vi "ICRA2024没有ratio控制只有轨迹跟踪.vi"() -> ()   [LabVIEW 2018]
doc: "Demonstrates the use of the Network Streams functions to send LED status to the myRIO target."
uses:
  <vilib>/Utility/file.llb/Read Delimited Spreadsheet (string).vi
  <vilib>/ErrorRing/Error Ring.xnode
  <vilib>/vision/NI_Vision_Development_Module.lvlib
panel:
  out "轨迹跟踪点数":i32[](array[numeric])
  out "数据总":dbl[][](array[numeric])
  out "时间T":i32[](array[numeric])
  out "运动方向":sgl[](array[numeric])
  out "aspectratio":dbl[](array[numeric])
  in  "轨迹打开":bool
  out "实际纵坐标":sgl
  out "实际横坐标":sgl
  out "方向d1":sgl
  out "轨迹跟踪点数":i32
  out "目标点y":dbl
  out "目标点x":dbl
  out "b":dbl[](array[numeric])
  in  "pp":dbl
  out "与目标点的距离":sgl
  in  "guiji":path=path "D:/lyz/ICRA2024-YuezhenLiu/small_myRIO_Helmholtz - 1111ke777/zgj轨迹跟踪只有20个点.txt" caption="call7-8"
  out "裁剪后的二值图":T1(plugin-control)
  in  "布尔":bool
  in  "ribbon磁场开关":bool=TRUE
  out "面积":sgl
  out "field ratio":sgl=4.0
  out "时间":i32
  out "aspect ratio":dbl
  out "D2":i32
  out "D1":i32
  out "二值图":T1(plugin-control)
  in  "Search Rect (entire image)":T2={"Left"=200, "Top"=120, "Right"=2000, "Bottom"=1920, "Rotation"=0.0} {"Rotation" format="%.2f"; "Left" scale=0.0..1024.0; "Right" scale=0.0..1024.0}
  out "备用的椭圆角度":sgl
  in  "Number of Erosion":i32=10
  out "Image 7":T1(plugin-control)
  in  "Acquisition Control::Acquisition Frame Rate":dbl=19.50304412841797 min=1.4211589097976685 max=44.94382095336914
  out "Stopped":bool
  in  "Stop (F) 2":bool caption="Stop (F)"
  out "Objects 2":T3(array[cluster]) {"Aspect Ratio" format="%.2f"; "Orientation" format="%.2f"; "Area" format="%.2f"; "Object Center"."Y" format="%.2f"; "Object Center"."X" format="%.2f"}
  in  "Settings 2":T4={"Objects"=0, "Threshold"=128, "Reject Border"=FALSE, "Fill Holes"=FALSE, "Min Object Size"=FALSE, "Min Size"=20000, "Max Object Size"=FALSE, "Max Size"=100, "Show Search Area"=FALSE, "Show Center"=TRUE, "Show Bounding Box"=TRUE} {"Objects" items=["Bright Objects", "Dark Objects"]; "Threshold" min=1 max=999999999 step=1; "Max Size" min=1 max=999999999 step=1; "Min Size" min=1 max=999999999 step=1}
  in  "Range 2":cluster{"Lower value":sgl, "Upper value":sgl}={"Lower value"=0.0, "Upper value"=230.0} {"Upper value" format="%.2f"; "Lower value" format="%.2f"}
  in  "Pause":bool
  out "Array":dbl[](array[numeric])
  in  "Parameter Settings":T5(tab)=enum."Ribbon Oscillating Field" caption="Field Types"
  in  "fg":dbl
  in  "pg":dbl
  in  "dg":dbl
  in  "Ag":dbl
  in  "AoOF":dbl
  in  "fo":sgl
  in  "do":sgl
  in  "oo":sgl
  in  "po":sgl
  in  "cc":sgl
  in  "pc":sgl
  in  "wc":sgl
  in  "dc":sgl
  in  "Ac":dbl
  in  "pr":sgl
  in  "Ar":dbl=8.0
  in  "wr":sgl=18.0
  in  "dr":sgl
  in  "Dis phase step":dbl
  in  "Dis phase frequency (Hz)":dbl
  in  "Dis tumbling frequency (Hz)":dbl
  in  "Dis strength(mT)":dbl
  in  "Swa strength (mT)":dbl
  in  "Swa frequency (Hz)":dbl
  in  "Swa pitch angle (deg)":dbl
  in  "Swa direction angle (deg)":dbl
  in  "Swa ratio":dbl=1.0
  in  "Pitch Angle (rotating around Constant, deg)":dbl
  in  "Ratio (A/C)":sgl=4.0
  in  "Direction Angle (deg)":sgl
  in  "Pitch Angle (rotating around Origin, deg)":sgl
  in  "Frequency (Hz)":sgl=10.0
  in  "Strength (mT)":dbl=10.0
  in  "Ar 2":dbl=5.0 caption="Ar"
  in  "ratio":sgl=1.0
  in  "运动方向":sgl
  in  "长轴方向":sgl
  in  "wr  2":sgl=8.0
  in  "速度大小":sgl
  out "Numeric 5":i32
  in  "Stop":bool
  out "error out":errorcluster
  in  "Target IP Address":string="172.22.11.2"
  # "Overview: Magnetic field calculation, and send parameters to myRIO\nInstructions:\n1. Verify the value of Target IP Address. Set Visa resource name.\n2. Ensure RT Main.vi is already running. \n3. Run this VI. Set parameters of magnetic field."
  # "Strength (mT)"
  # "Pitch Angle (deg)"
  # "Direction Angle (deg)"
  # "Frequency (Hz)"
  # "Strength (mT)"
  # "Oscilation Frequency (Hz)"
  # "Oscilation Angle (deg)"
  # "Pitch Angle (deg)"
  # "Direction Angle (deg)"
  # "Strength (mT)"
  # "Frequency (Hz)"
  # "Pitch Angle (deg)"
  # "Direction Angle (deg)"
  # "Conical Angle (deg)"
  # "Strength (mT)"
  # "Frequency (Hz)"
  # "Pitch Angle (deg)"
  # "Direction Angle (deg)"
  # "Strength (mT)"
  # "Tumbling Frequency (Hz)"
  # "Phase Frequency (Hz)"
  # "Phase Step"
  # "Strength (mT)"
  # "Frequency (Hz)"
  # "Pitch Angle (deg)"
  # "Direction Angle (deg)"
  # "Ratio"
  # "Strength (mT)"
  # "Frequency (Hz)"
  # "Ratio (A/C)"
  # "Direction Angle (deg)"
  # "Pitch Angle (rotating around Origin, deg)"
  # "Pitch Angle (rotating around Constant, deg)"
  # "Strength (mT)"
  # "Frequency (Hz)"
  # "Pitch Angle  (deg)"
  # "longaxis"
  # "Direction Angle (deg)"
  # "ratio (l/s)"
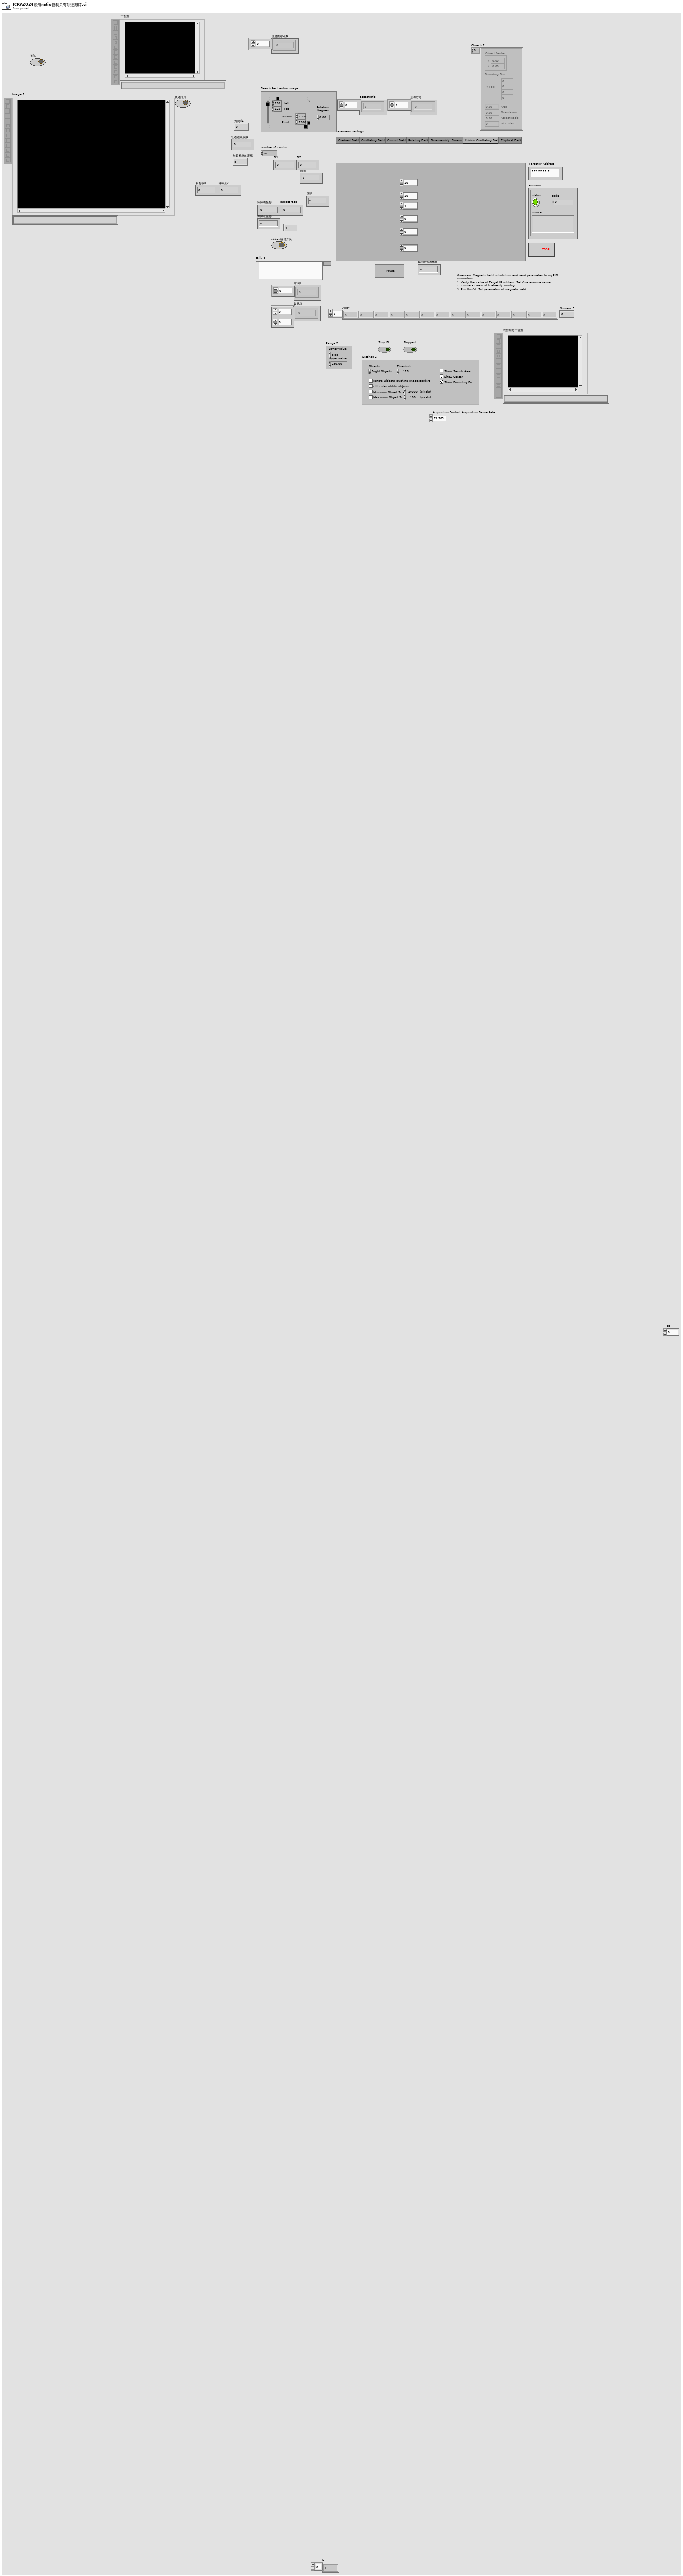
[diagram p1: front panel]
types:
  T1 = typedef "IMAQ Image.ctl" = refnum<image>
  T2 = typedef "IMAQ Rectangle" = cluster{"Left":i32, "Top":i32, "Right":i32, "Bottom":i32, "Rotation":dbl}
  T3 = cluster{"Object Center":cluster{"X":sgl, "Y":sgl}, "Bounding Box":cluster{"X Left":i32, "Y Top":i32, "X Right":i32, "Y Bottom":i32}, "Area":sgl, "Orientation":sgl, "Aspect Ratio":sgl, "Nb Holes":i32}[]
  T4 = cluster{"Objects":u16, "Threshold":i32, "Reject Border":bool, "Fill Holes":bool, "Min Object Size":bool, "Min Size":i32, "Max Object Size":bool, "Max Size":i32, "Show Search Area":bool, "Show Center":bool, "Show Bounding Box":bool}
  T5 = enum32{"Gradient Field ", "Oscillating Field", "Conical Field", "Rotating Field", "Disassembly", "Swarm", "Ribbon Oscillating Field", "Elliptical Field"}
  T6 = typedef "Image Type" = u32
  T7 = cluster{"Objects[0]":cluster{"Object Center":cluster{"X":sgl, "Y":sgl}, "Bounding Box":cluster{"X Left":i32, "Y Top":i32, "X Right":i32, "Y Bottom":i32}, "Area":sgl, "Orientation":sgl, "Aspect Ratio":sgl, "Nb Holes":i32}, "Objects[1]":cluster{"Object Center":cluster{"X":sgl, "Y":sgl}, "Bounding Box":cluster{"X Left":i32, "Y Top":i32, "X Right":i32, "Y Bottom":i32}, "Area":sgl, "Orientation":sgl, "Aspect Ratio":sgl, "Nb Holes":i32}, "Objects[2]":cluster{"Object Center":cluster{"X":sgl, "Y":sgl}, "Bounding Box":cluster{"X Left":i32, "Y Top":i32, "X Right":i32, "Y Bottom":i32}, "Area":sgl, "Orientation":sgl, "Aspect Ratio":sgl, "Nb Holes":i32}, "Objects[3]":cluster{"Object Center":cluster{"X":sgl, "Y":sgl}, "Bounding Box":cluster{"X Left":i32, "Y Top":i32, "X Right":i32, "Y Bottom":i32}, "Area":sgl, "Orientation":sgl, "Aspect Ratio":sgl, "Nb Holes":i32}, "Objects[4]":cluster{"Object Center":cluster{"X":sgl, "Y":sgl}, "Bounding Box":cluster{"X Left":i32, "Y Top":i32, "X Right":i32, "Y Bottom":i32}, "Area":sgl, "Orientation":sgl, "Aspect Ratio":sgl, "Nb Holes":i32}, "Objects[5]":cluster{"Object Center":cluster{"X":sgl, "Y":sgl}, "Bounding Box":cluster{"X Left":i32, "Y Top":i32, "X Right":i32, "Y Bottom":i32}, "Area":sgl, "Orientation":sgl, "Aspect Ratio":sgl, "Nb Holes":i32}, "Objects[6]":cluster{"Object Center":cluster{"X":sgl, "Y":sgl}, "Bounding Box":cluster{"X Left":i32, "Y Top":i32, "X Right":i32, "Y Bottom":i32}, "Area":sgl, "Orientation":sgl, "Aspect Ratio":sgl, "Nb Holes":i32}, "Objects[7]":cluster{"Object Center":cluster{"X":sgl, "Y":sgl}, "Bounding Box":cluster{"X Left":i32, "Y Top":i32, "X Right":i32, "Y Bottom":i32}, "Area":sgl, "Orientation":sgl, "Aspect Ratio":sgl, "Nb Holes":i32}, "Objects[8]":cluster{"Object Center":cluster{"X":sgl, "Y":sgl}, "Bounding Box":cluster{"X Left":i32, "Y Top":i32, "X Right":i32, "Y Bottom":i32}, "Area":sgl, "Orientation":sgl, "Aspect Ratio":sgl, "Nb Holes":i32}}
  T8 = cluster{"Object Center":cluster{"X":sgl, "Y":sgl}, "Bounding Box":cluster{"X Left":i32, "Y Top":i32, "X Right":i32, "Y Bottom":i32}, "Area":sgl, "Orientation":sgl, "Aspect Ratio":sgl, "Nb Holes":i32}
  T9 = cluster{"X Left":i32, "Y Top":i32, "X Right":i32, "Y Bottom":i32}
  T10 = typedef "ROI Descriptor" = cluster{"Global Rectangle":i32[], "Contours":cluster{"ID":enum32{"External", "Internal"}, "Type":u32, "Coordinates":i32[]}[]}
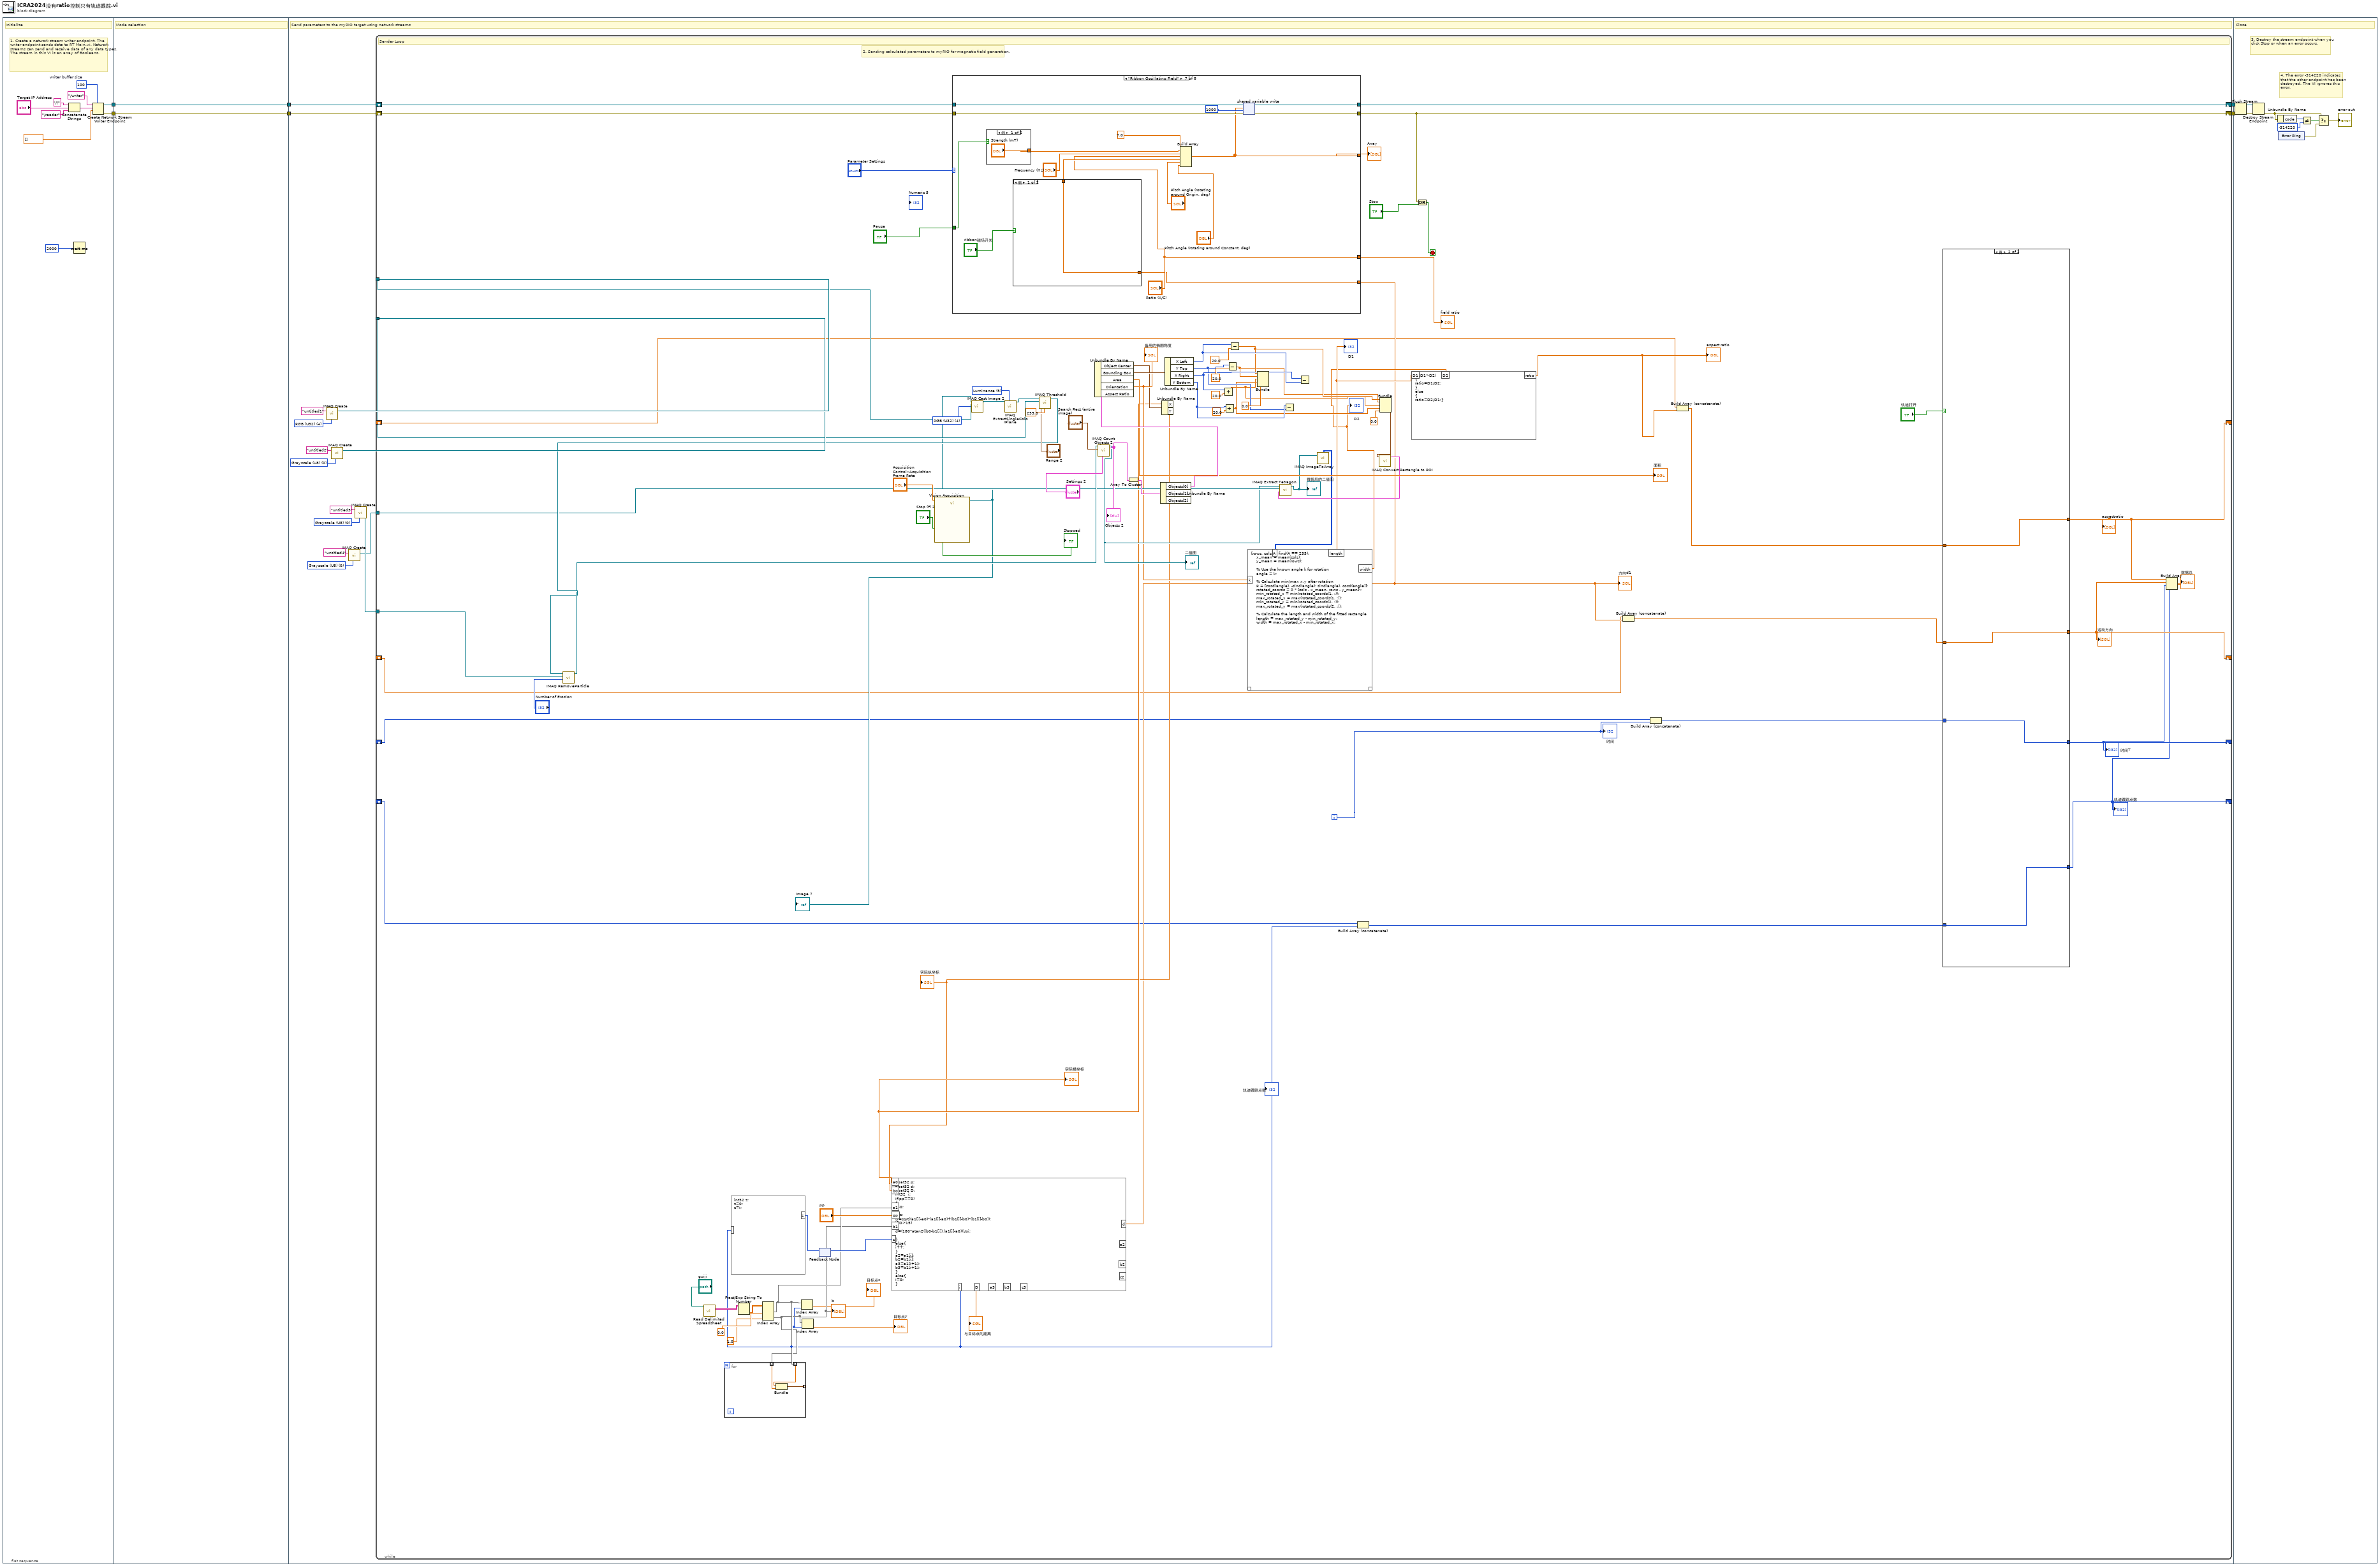
[diagram p0: block diagram]
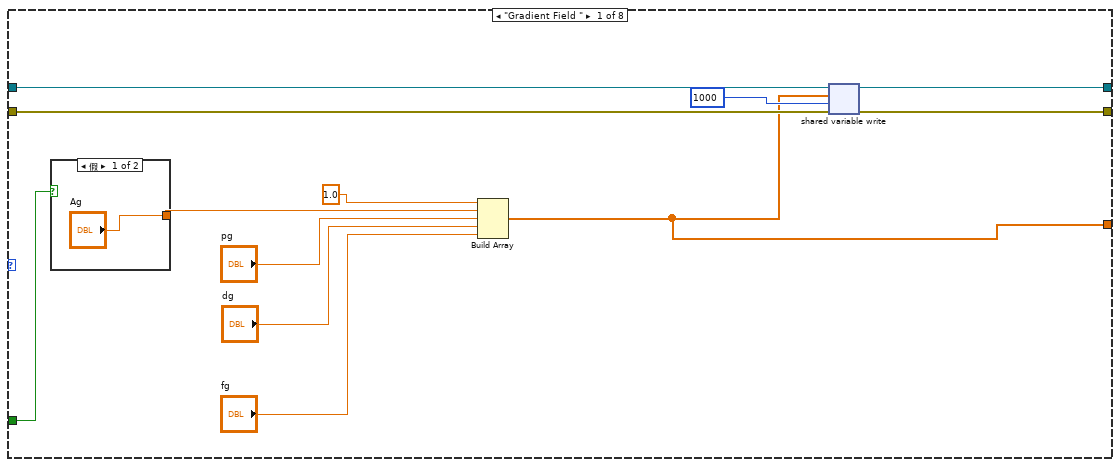
[diagram p3: hidden frame]
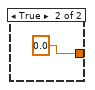
[diagram p4: hidden frame]
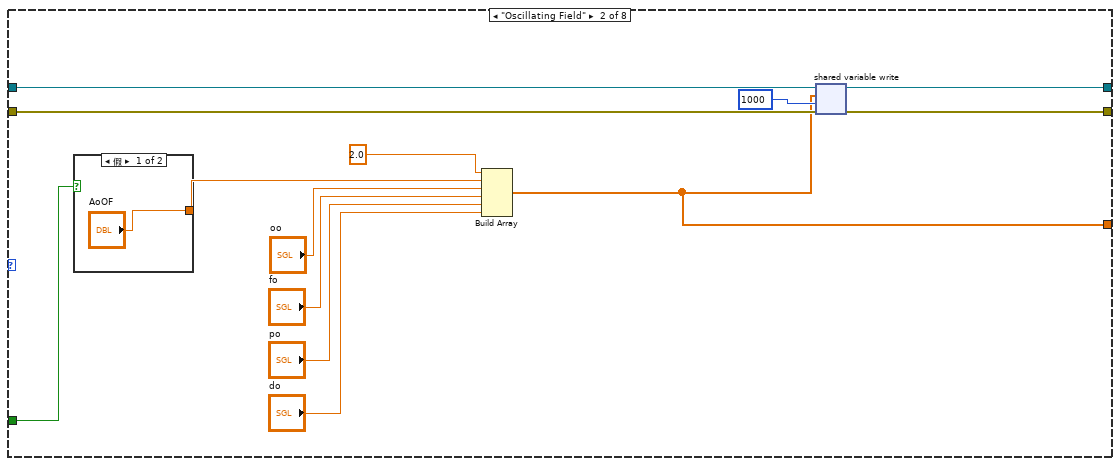
[diagram p5: hidden frame]
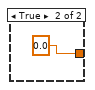
[diagram p6: hidden frame]
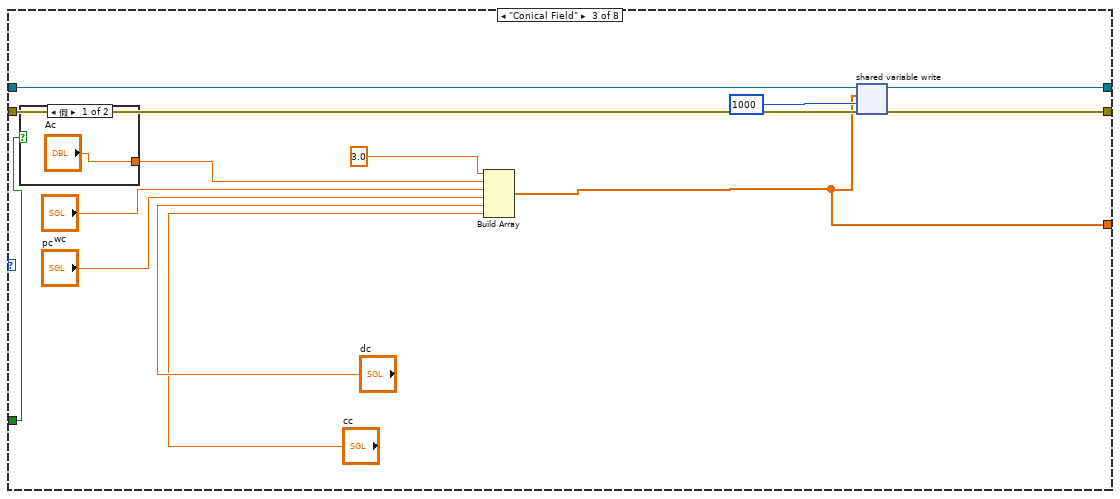
[diagram p7: hidden frame]
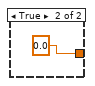
[diagram p8: hidden frame]
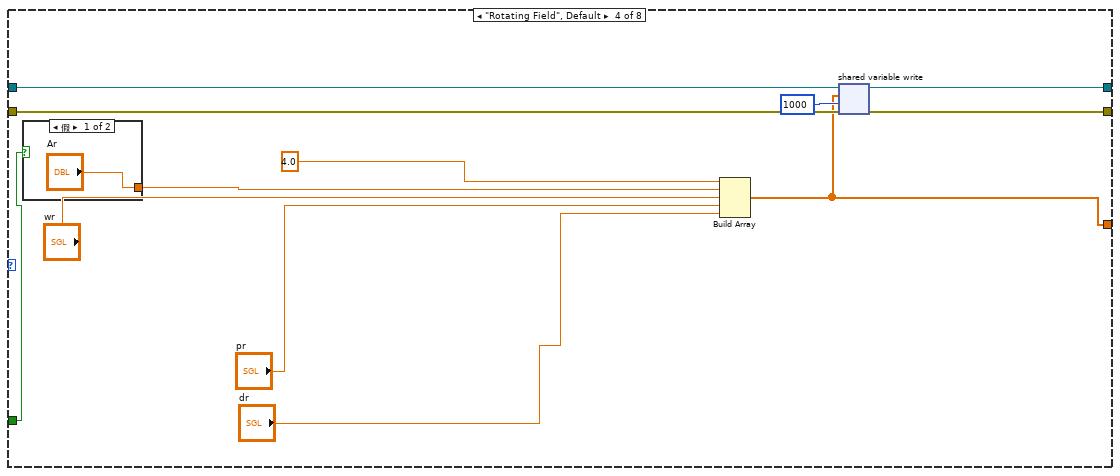
[diagram p9: hidden frame]
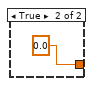
[diagram p10: hidden frame]
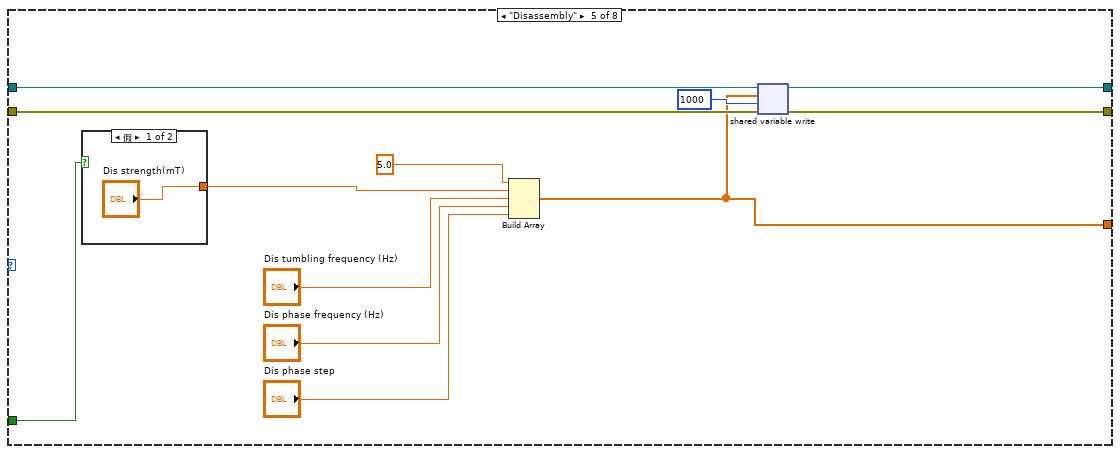
[diagram p11: hidden frame]
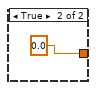
[diagram p12: hidden frame]
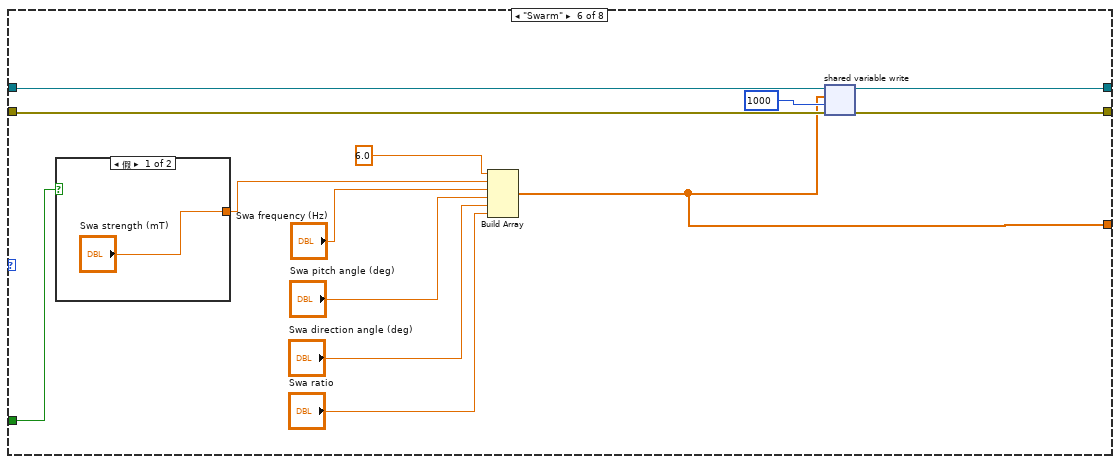
[diagram p13: hidden frame]
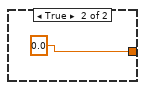
[diagram p14: hidden frame]
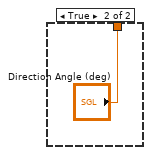
[diagram p15: hidden frame]
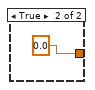
[diagram p16: hidden frame]
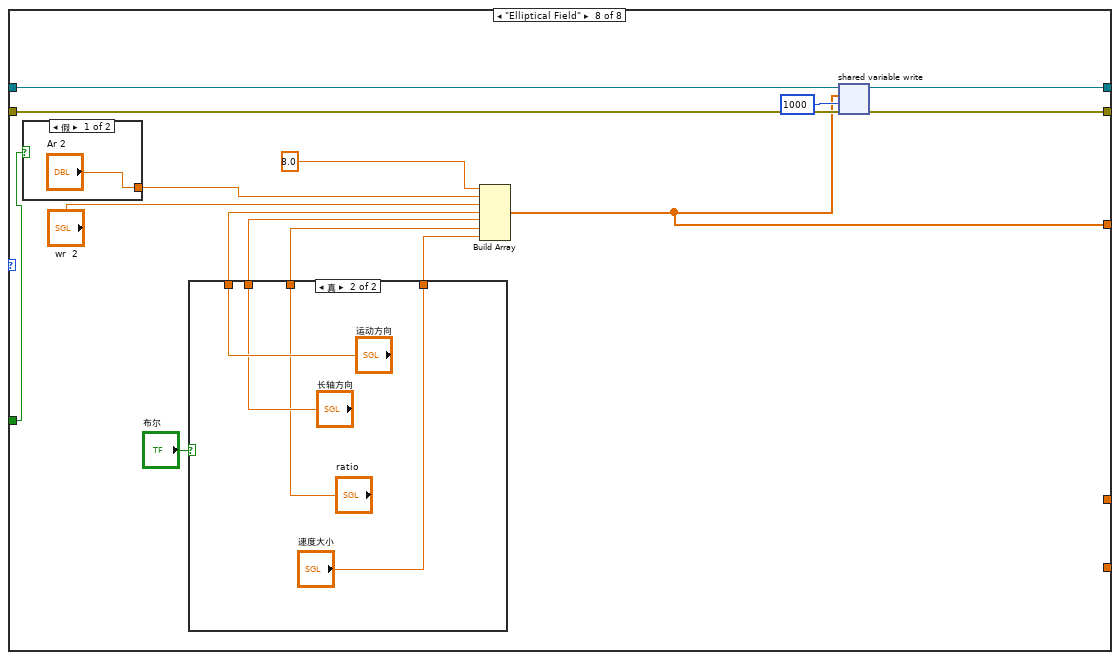
[diagram p17: hidden frame]
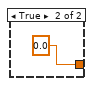
[diagram p19: hidden frame]
diagram:
  n1 = flat-sequence {
    tunnel: [w11] -> w2
    tunnel: [w10] -> w1
    tunnel: [w18] -> w4
    tunnel: [w17] -> w3
    tunnel: w1 -> [w17]
    tunnel: w2 -> [w18]
    tunnel: [w32] -> w6
    tunnel: w4 -> [w34]
    tunnel: [w31] -> w5
    tunnel: w3 -> [w33]
    tunnel: w6 -> [w269]
    tunnel: w5 -> [w266]
    frame #0 {
      w9 = 100  # writer buffer size
      # "1. Create a network stream writer endpoint. The writer endpoint sends data to RT Main.vi. Network streams can send and receive data of any data types. The stream in this VI is an array of Booleans."
      # "Initialize"
      n2 = Concatenate Strings("//", "Target IP Address", "/reader") -> (w16:string)
      n3 = Wait (ms)(milliseconds to wait=2000) -> ()  [unwired: 1 out]
      n4 = Create Network Stream Writer Endpoint(7:w9, 9:dbl[] [], 10:w16, 11:"/writer" ("reader name")) -> (0:w10:errorcluster, 3:w11:refnum<k21>)  [unwired: 3 in]
    }
    frame #1 {
      # "Mode selection"
    }
    frame #2 {
      w20 = T6 0 items=["Grayscale (U8)", "Grayscale (I16)", "Grayscale (SGL)", "Complex (CSG)", "RGB (U32)", "HSL (U32)", "RGB (U64)", "Grayscale (U16)"] ("Image Type")
      w23 = T6 0 items=["Grayscale (U8)", "Grayscale (I16)", "Grayscale (SGL)", "Complex (CSG)", "RGB (U32)", "HSL (U32)", "RGB (U64)", "Grayscale (U16)"] ("Image Type")
      w27 = T6 0 items=["Grayscale (U8)", "Grayscale (I16)", "Grayscale (SGL)", "Complex (CSG)", "RGB (U32)", "HSL (U32)", "RGB (U64)", "Grayscale (U16)"] ("Image Type")
      w29 = T6 4 items=["Grayscale (U8)", "Grayscale (I16)", "Grayscale (SGL)", "Complex (CSG)", "RGB (U32)", "HSL (U32)", "RGB (U64)", "Grayscale (U16)"] ("Image Type")
      # "Send parameters to the myRIO target using network streams"
      n5 = call "IMAQ Create"("Image Name"="untitled1", "Image Type"=w29) -> ("New Image"=w26:T1)  [unwired: 3 in, 1 out]
      n6 = call "IMAQ Create"("Image Name"="untitled2", "Image Type"=w27) -> ("New Image"=w25:T1)  [unwired: 3 in, 1 out]
      n7 = call "IMAQ Create"("Image Name"="untitled4", "Image Type"=w20) -> ("New Image"=w19:T1)  [unwired: 3 in, 1 out]
      n8 = call "IMAQ Create"("Image Name"="untitled3", "Image Type"=w23) -> ("New Image"=w22:T1)  [unwired: 3 in, 1 out]
      n9 = while {
        shift-right: [w120] -> w31
        shift-left: w33 -> [w122]
        shift-right: [w121] -> w32
        shift-left: w34 -> [w123]
        tunnel: w25 -> [w111]
        tunnel: w26 -> [w106]
        tunnel: w22 -> [w95]
        tunnel: w19 -> [w84]
        shift-right: [w41] -> _
        shift-left: _ -> [w49]
        shift-right: [w42] -> _
        shift-left: _ -> [w46]
        shift-right: [w40] -> _
        shift-left: _ -> [w43]
        shift-right: [w36] -> _
        shift-left: _ -> [w35]
        i -> [w45]
        stop <- w110 stop-if-true
        w105 = T6 4 items=["Grayscale (U8)", "Grayscale (I16)", "Grayscale (SGL)", "Complex (CSG)", "RGB (U32)", "HSL (U32)", "RGB (U64)", "Grayscale (U16)"] ("Image Type")
        w116 = 5 items=["Red", "Green", "Blue", "Hue", "Saturation", "Luminance", "Value", "Intensity"] ("Color Plane")
        # "2. Sending calculated parameters to myRIO for magnetic field generation."
        # "Sender Loop"
        n10 = call-poly <vilib>:"Read Delimited Spreadsheet.vi"("file path (dialog if empty)"="guiji") -> ("all rows"=w68:string[][])  [unwired: 9 in, 5 out]
        n11 = Fract/Exp String To Number(string=w68) -> (number=w67:dbl[][])  [unwired: 3 in, 1 out]
        n12 = Index Array(array=w67, index (col) #1=0.0, index (col) #2=1.0) -> (element #1=w60:dbl[], element #2=w59:dbl[])  [unwired: 2 in]
        "b" <- w59
        n13 = for {
          tunnel: w60 -> [w131] mode=indexing
          tunnel: w59 -> [w130] mode=indexing
          tunnel: [w129] -> _ mode=indexing
          n14 = Bundle("String"=w131, "String"=w130) -> (w129:cluster{"String":dbl, "String":dbl})  [unwired: 1 in]
        }
        n15 = feedback #1() -> (w63:i32)  [unwired: 1 in]
        n16 = call "Vision Acquisition"("Acquisition Control::Acquisition Frame Rate"="Acquisition Control::Acquisition Frame Rate", "Stop (F)"="Stop (F) 2") -> ("Image Out"=w70:T1, "Stopped"=→"Stopped":bool)  [unwired: 23 in, 1 out]
        "Image 7" <- w70
        n17 = call "IMAQ Cast Image 2"("Image Src"=w70, "Image Dst"=w106, "Image Type"=w105) -> ("Image Dst Out"=w107:T1)  [unwired: 11 in, 1 out]
        n18 = call "IMAQ ExtractSingleColorPlane"("Color Plane"=w116, "Image Src"=w107) -> ("Image Dst Out"=w53:T1)  [unwired: 8 in, 1 out]
        n19 = call "IMAQ Threshold"("Replace Value"=sgl 255.0, "Range"="Range 2", "Image Dst"=w111, "Image Src"=w53) -> ("Image Dst Out"=w96:T1)  [unwired: 6 in, 1 out]
        n20 = call "IMAQ RemoveParticle"("Number of Erosion"="Number of Erosion", "Image Dst"=w95, "Image Src"=w96) -> ("Image Dst Out"=w89:T1)  [unwired: 7 in, 1 out]
        n21 = call "IMAQ Count Objects 2"("Settings"="Settings 2", "Search Rect (entire image)"="Search Rect (entire image)", "Image"=w89) -> ("Image Out"=w83:T1, "Objects"=w112:T3)  [unwired: 4 in, 3 out]
        "Objects 2" <- w112
        "二值图" <- w83
        n22 = Array To Cluster(array=w112) -> (cluster=w98:T7)
        n23 = Unbundle By Name(w98) -> ("Objects[0]"=w97:T8)  [unwired: 2 out]
        n24 = Unbundle By Name(w97) -> ("Object Center"=w56:cluster{"X":sgl, "Y":sgl}, "Bounding Box"=w104:T9, "Area"=→"面积":sgl, "Orientation"=w71:sgl)  [unwired: 1 out]
        "备用的椭圆角度" <- w71
        n25 = Unbundle By Name(w56) -> ("X"=w55:sgl, "Y"=w54:sgl)
        "实际横坐标" <- w55
        "实际纵坐标" <- w54
        n26 = formula code="float32 p;\nfloat32 d;\nfloat32 D;\nint32  i;\nif(pp==0)\n{\ni=0;\n\ni=z;\nD=sqrt((a1[i]-a0)*(a1[i]-a0)+(b1[i]-b0)*(b1[i]-b0));\nif(D>15)\n{\nd=(180*atan2((b0-b1[i]),(a1[i]-a0)))/pi;\n\n}\nelse{\ni++;\n}\na2=a1[i];\nb2=b1[i];\na3=a1[i+1];\nb3=b1[i+1];\n}\nelse{\ni=0;\n}"("a0"=w55, "b0"=w54, "a1"=w60, "b1"=w59, "z"=w63, "pp"="pp") -> ("i"=w38:i32, "D"=→"与目标点的距离":sgl, "d"=w51:sgl)  [unwired: 6 out]
        "轨迹跟踪点数" <- w38
        "方向d1" <- w51
        n27 = formula code="int32 z;\nz=0;\nz=i;"("i"=w38) -> ("z"=w64:i32)
        n28 = Index Array(array=w60, index=w38) -> (element=→"目标点x":dbl)
        n29 = Index Array(array=w59, index=w38) -> (element=→"目标点y":dbl)
        n30 = feedback-in #1(w64) -> ()
        n31 = case shown="\"Ribbon Oscillating Field\"" "Parameter Settings" {
          tunnel: w123 -> [w142 w157 w172 w186 w200 w214 w234 w252]
          tunnel: w122 -> [w139 w156 w171 w185 w198 w213 w232 w251]
          tunnel: [w141 w155 w169 w184 w199 w212 w233 w250] -> w121
          tunnel: [w140 w154 w170 w183 w197 w211 w231 w249] -> w120
          tunnel: [w135 w148 w163 w178 w191 w206 w229 w244] -> w119
          tunnel: "Pause" -> [w133 w146 w161 w176 w190 w205 w226 w242]
          tunnel: [_ _ _ _ _ _ "Ratio (A/C)" _] -> w86
          tunnel: w51 -> [_ _ _ _ _ _ w219 _]
          frame "Gradient Field " {
            n32 = case shown="假" w133 {
              tunnel: ["Ag" 0.0] -> w134
              frame False {
              }
              frame True {
              }
            }
            n33 = Build Array(1.0, w134, "pg", "dg", "fg") -> (w135:dbl[])
            n34 = shared-variable-write(w142, w139, w135, 1000 ("timeout ms (-1)")) -> (w141:refnum<k21>, w140:errorcluster)  [unwired: 1 out]
          }
          frame "Oscillating Field" {
            n35 = case shown="假" w146 {
              tunnel: ["AoOF" 0.0] -> w147
              frame False {
              }
              frame True {
              }
            }
            n36 = Build Array(2.0, w147, "oo", "fo", "po", "do") -> (w148:dbl[])
            n37 = shared-variable-write(w157, w156, w148, 1000 ("timeout ms (-1)")) -> (w155:refnum<k21>, w154:errorcluster)  [unwired: 1 out]
          }
          frame "Conical Field" {
            # "FG"
            n38 = case shown="假" w161 {
              tunnel: ["Ac" 0.0] -> w162
              frame False {
              }
              frame True {
              }
            }
            n39 = Build Array(3.0, w162, "wc", "pc", "dc", "cc") -> (w163:dbl[])
            n40 = shared-variable-write(w172, w171, w163, 1000 ("timeout ms (-1)")) -> (w169:refnum<k21>, w170:errorcluster)  [unwired: 1 out]
          }
          frame "Rotating Field", Default {
            n41 = case shown="假" w176 {
              tunnel: ["Ar" 0.0] -> w177
              frame False {
              }
              frame True {
              }
            }
            n42 = Build Array(4.0, w177, "wr", "pr", "dr") -> (w178:dbl[])
            n43 = shared-variable-write(w186, w185, w178, 1000 ("timeout ms (-1)")) -> (w184:refnum<k21>, w183:errorcluster)  [unwired: 1 out]
          }
          frame "Disassembly" {
            n44 = case shown="假" w190 {
              tunnel: ["Dis strength(mT)" 0.0] -> w195
              frame False {
              }
              frame True {
              }
            }
            n45 = Build Array(5.0, w195, "Dis tumbling frequency (Hz)", "Dis phase frequency (Hz)", "Dis phase step") -> (w191:dbl[])
            n46 = shared-variable-write(w200, w198, w191, 1000 ("timeout ms (-1)")) -> (w199:refnum<k21>, w197:errorcluster)  [unwired: 1 out]
          }
          frame "Swarm" {
            n47 = case shown="假" w205 {
              tunnel: ["Swa strength (mT)" 0.0] -> w204
              frame False {
              }
              frame True {
              }
            }
            n48 = Build Array(6.0, w204, "Swa frequency (Hz)", "Swa pitch angle (deg)", "Swa direction angle (deg)", "Swa ratio") -> (w206:dbl[])
            n49 = shared-variable-write(w214, w213, w206, 1000 ("timeout ms (-1)")) -> (w212:refnum<k21>, w211:errorcluster)  [unwired: 1 out]
          }
          frame "Ribbon Oscillating Field" {
            n50 = case shown="假" w226 {
              tunnel: ["Strength (mT)" 0.0] -> w225
              frame False {
              }
              frame True {
              }
            }
            n51 = case shown="假" "ribbon磁场开关" {
              tunnel: [w235 "Direction Angle (deg)"] -> w222
              tunnel: w219 -> [w235 _]
              frame False {
              }
              frame True {
              }
            }
            n52 = Build Array(7.0, w225, "Frequency (Hz)", "Ratio (A/C)", w222, "Pitch Angle (rotating around Origin, deg)", "Pitch Angle (rotating around Constant, deg)") -> (w229:dbl[])
            n53 = shared-variable-write(w234, w232, w229, 1000 ("timeout ms (-1)")) -> (w233:refnum<k21>, w231:errorcluster)  [unwired: 1 out]
          }
          frame "Elliptical Field" {
            n54 = case shown="假" w242 {
              tunnel: ["Ar 2" 0.0] -> w243
              frame False {
              }
              frame True {
              }
            }
            n55 = case shown="真" "布尔" {
              tunnel: [_ "运动方向"] -> w247
              tunnel: [_ "长轴方向"] -> w246
              tunnel: [_ "ratio"] -> w241
              tunnel: [_ "速度大小"] -> w240
              frame False {
              }
              frame True {
              }
            }
            n56 = Build Array(8.0, w243, "wr  2", w247, w246, w241, w240) -> (w244:dbl[])
            n57 = shared-variable-write(w252, w251, w244, 1000 ("timeout ms (-1)")) -> (w250:refnum<k21>, w249:errorcluster)  [unwired: 1 out]
          }
        }
        "Array" <- w119
        "field ratio" <- w86
        n58 = Unbundle By Name(w104) -> ("X Left"=w91:i32, "Y Top"=w87:i32, "X Right"=w92:i32, "Y Bottom"=w88:i32)
        n59 = Add(x=w92, y=20.0) -> (x+y=w78:dbl)
        n60 = Add(x=w88, y=20.0) -> (x+y=w77:dbl)
        n61 = Subtract(x=w87, y=20.0) -> (x-y=w79:dbl)
        n62 = Subtract(x=w91, y=20.0) -> (x-y=w80:dbl)
        n63 = Bundle(w80, w79, w78, w77, 0.0) -> ()  [unwired: 1 in, 1 out]
        n64 = Subtract(x=w88, y=w87) -> ()  [unwired: 1 out]
        n65 = Subtract(x=w92, y=w91) -> ()  [unwired: 1 out]
        n66 = Build Array (concatenate)(w35, w38) -> (w37:i32[])
        n67 = Bundle(w80, w79, w78, w77, 0.0) -> (w75:cluster{dbl, dbl, dbl, dbl, dbl})  [unwired: 1 in]
        n68 = call "IMAQ Convert Rectangle to ROI"("Rectangle"=w75) -> ("ROI Descriptor"=w81:T10)  [unwired: 8 in, 1 out]
        n69 = call-poly "IMAQ Extract Tetragon"("ROI Descriptor"=w81, "Image Dst"=w84, "Image Src"=w83) -> ("Image Dst Out"=w82:T1)  [unwired: 7 in, 1 out]
        "裁剪后的二值图" <- w82
        n70 = call "IMAQ ImageToArray"("Image"=w82) -> ("Image Pixels (U8)"=w74:u8[][])  [unwired: 3 in, 4 out]
        n71 = script code="[rows, cols] = find(A == 255);\n    x_mean = mean(cols);\n    y_mean = mean(rows);\n\n    % Use the known angle k for rotation\n    angle = k;\n\n    % Calculate min/max x,y after rotation\n    R = [cosd(angle), -sind(angle); sind(angle), cosd(angle)];\n    rotated_coords = R * [cols - x_mean, rows - y_mean]';\n    min_rotated_x = min(rotated_coords(1, :));\n    max_rotated_x = max(rotated_coords(1, :));\n    min_rotated_y = min(rotated_coords(2, :));\n    max_rotated_y = max(rotated_coords(2, :));\n\n    % Calculate the length and width of the fitted rectangle\n    length = max_rotated_y - min_rotated_y;\n    width = max_rotated_x - min_rotated_x;"("A"=w74, "k"=w71) -> ("length"=w73:dbl, "width"=w72:dbl)  [unwired: 1 in, 1 out]
        "D1" <- w73
        "D2" <- w72
        n72 = formula code="if (D1>D2)\n{\nratio=D1/D2;\n}\nelse\n{\nratio=D2/D1;}"("D1"=w73, "D2"=w72) -> ("ratio"=w48:dbl)
        "aspect ratio" <- w48
        n73 = Or(x=w120, y="Stop") -> (x .or. y?=w110:bool)
        n74 = Build Array (concatenate)(w49, w51) -> (w50:sgl[])
        n75 = Build Array (concatenate)(w43, w45) -> (w44:i32[])
        n76 = Build Array (concatenate)(w46, w48) -> (w47:dbl[])
        n77 = case shown="真" "轨迹打开" {
          tunnel: [_ w128] -> w41
          tunnel: w50 -> [_ w128]
          tunnel: [_ w127] -> w42
          tunnel: w47 -> [_ w127]
          tunnel: [_ w126] -> w40
          tunnel: w44 -> [_ w126]
          tunnel: [_ w125] -> w36
          tunnel: w37 -> [_ w125]
          frame False {
          }
          frame True {
          }
        }
        "aspectratio" <- w42
        "运动方向" <- w41
        "时间T" <- w40
        "轨迹跟踪点数" <- w36
        n78 = Build Array(w42, w41, w40, w36) -> (→"数据总":dbl[][])
        "时间" <- w45
      }
    }
    frame #3 {
      # "4. The error -314220 indicates that the other endpoint has been destroyed. The VI ignores this error."
      # "3. Destroy the stream endpoint when you click Stop or when an error occurs."
      # "Close"
      n79 = Flush Stream(8:w266, 11:w269) -> (0:w267:errorcluster, 3:w268:refnum<k21>)  [unwired: 2 in, 1 out]
      n80 = Destroy Stream Endpoint(8:w267, 11:w268) -> (0:w261:errorcluster)
      n81 = Unbundle By Name(w261) -> ("code"=w265:i32)
      n82 = xnode "Error Ring"() -> ("错误输出"=w262:errorcluster)
      n83 = Not Equal?(x=w265, y=-314220) -> (x != y?=w263:bool)
      n84 = Select(t=w261, s=w263, f=w262) -> (s? t:f=→"error out":errorcluster)
    }
  }
